vi "delete_Empty String to Name.vi"(11 "Date":string) -> (3 "name":string)   [LabVIEW 2019, in "Logger.Error.lvclass"]
uses:
  Logger.Error.lvclass
  <vilib>/Utility/Data Type/NI_Data Type.lvlib
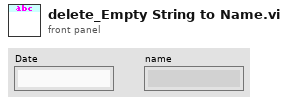
[diagram p1: front panel]
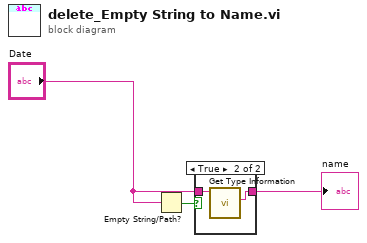
[diagram p0: block diagram]
diagram:
  n1 = Empty String/Path?(string/path="Date") -> (empty?=w2:bool)
  n2 = case shown="True" w2 {
    tunnel: "Date" -> [w4 w6]
    tunnel: [w4 w5] -> w3
    frame False {
    }
    frame True {
      n3 = call <vilib>:"Get Type Information.vi"("variant"=w6) -> ("name"=w5:string)  [unwired: 6 in, 4 out]
    }
  }
  "name" <- w3
